vi "滑移力检测.vi"() -> ()   [LabVIEW 2020]
uses:
  <vilib>/Utility/miscctls.llb/LVRowAndColumnTypeDef.ctl
  Global_Variable/Global.vi
  Global_Variable/A131258.vi
  Database/Global1.vi
  <vilib>/addons/database/Connection.llb/DB Tools Open Connec (String).vi
  <vilib>/addons/database/Connection.llb/Conn Execute.vi
  <vilib>/addons/database/Recordset.llb/Rec Fetch Recordset Data (R).vi
  <vilib>/Utility/config.llb/NI_LVConfig.lvlib
  <vilib>/addons/database/NI_Database_API.lvlib
panel:
  out "最大值下限":dbl format="%_4g"
  out "最大值上限":dbl format="%_4g"
  out "拉位移内最大压力(N)":dbl format="%_5g"
  out "压位移内最大压力(N)":dbl format="%_5g"
  out "上序状态显示":string
  out "上序状态":bool
  out "产品追溯码":string
  in  "质量报警":bool
  in  "设备缺料":bool
  in  "设备故障":bool
  out "USER_ID":string
  out "产品型号":string
  out "联机模式":string
  out "用户权限":string
  out "用户名":string
  in  "报表":string[][](table)=[["mm"], ["mm/s"]]
  in  "判定结果 3":bool[][](array[boolean])=[[TRUE]]
  out "拉力判定框内波动压力(N)":dbl format="%_5g"
  out "压力判定框内波动压力(N)":dbl format="%_5g"
  in  "选项卡控件 2":enum32{"滑移力曲线", "参数查看"}(tab)
  out "力位移曲线 3":cluster{dbl[], dbl[]}[](graph)
  out "压位移内最小压力(N)":dbl format="%_5g"
  out "拉位移内最小压力(N)":dbl format="%_5g"
  out "最小值上限":dbl format="%_4g"
  out "最小值下限":dbl format="%_4g"
  in  "产品型号":string(combo)
  in  "选项卡控件 3":enum32{"工位参数", "产品管理", "用户管理"}(tab)
  in  "启用最小值":bool
  in  "坐标轴参数":string[][](table)=[["mm"], ["mm/s"]]
  in  "判定框参数":string[][](table)=[["mm"], ["mm/s"]]
  in  "结果判定参数":string[][](table)=[["mm"], ["mm/s"]]
  in  "删除":bool
  in  "确定":bool
  in  "添加":bool
  in  "退出":bool
  in  "更新":bool
  in  "请输入添加的产品名称":string
  in  "请选择要删除的产品":string(combo)
  in  "进入用户管理":bool
  out "deviceid":string
  out "Fdeviceid":string
  out "codeid":string
  out "productid":string
  out "产品追溯码 2":string
  # "上序状态："
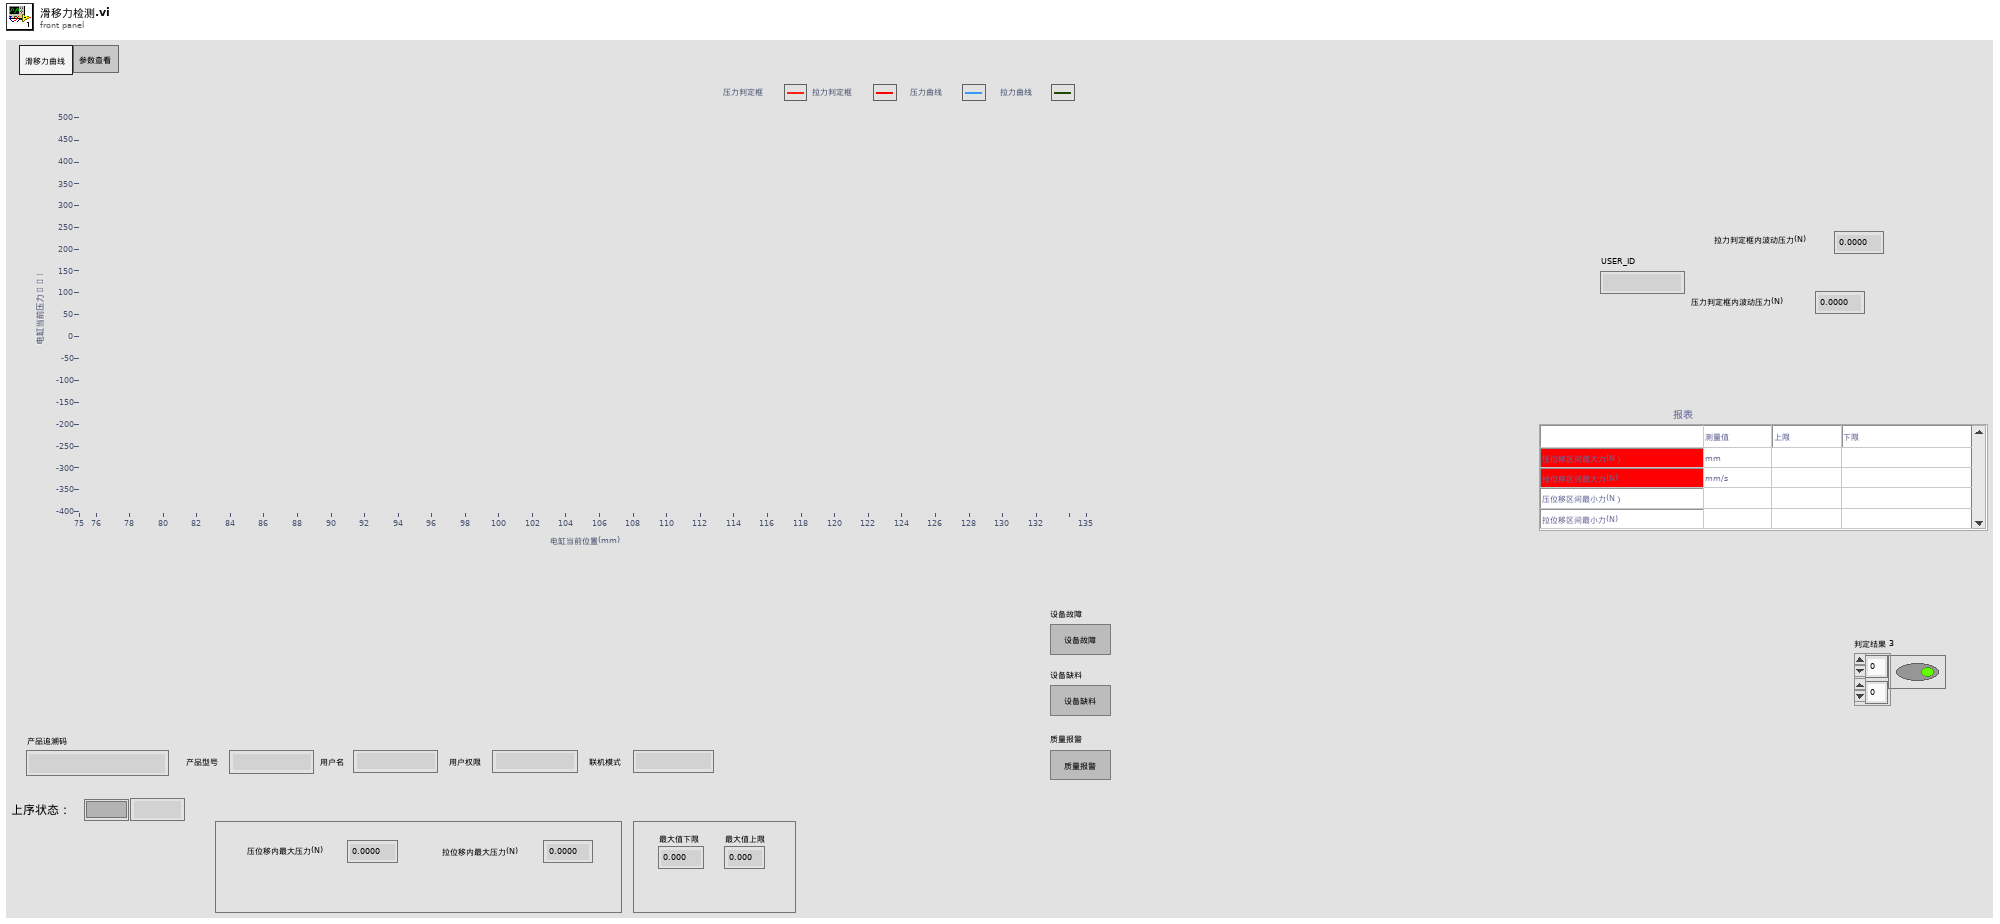
[diagram p1: front panel]
types:
  T1 = enum32{"Invalid", "Standard", "Closed", "Hidden", "Minimized", "Maximized"}
  T2 = typedef "LVRowAndColumnTypeDef.ctl" = cluster{"Row":i32, "Column":i32}
  T3 = cluster{"用户编号":string, "用户名":string, "用户密码(密文)":string, "用户权限":string}
  T4 = cluster{"设备名称":string, "用户名":string, "设备状态":enum16{"设备离线", "设备正常", "设备缺料", "设备故障", "质量报警"}, "附加信息":string}
  T5 = typedef "NI_LVConfig.lvlib/Config Data RefNum.ctl" = refnum<k1>
  T6 = cluster{"输入旋转位移":sgl, "电缸位移":sgl, "工装移载位移":sgl, "输入编码位移":sgl, "输入扭矩":sgl, "123":sgl, "拉压力":sgl, "吸收电流":sgl}
  T7 = cluster{"测试范围":cluster{"单位":string, "下限":dbl, "上限":dbl}, "压力测试最大值":cluster{"单位":string, "下限":dbl, "上限":dbl}, "拉力测试最大值":cluster{"单位":string, "下限":dbl, "上限":dbl}}
  T8 = cluster{"测试范围":cluster{"单位":string, "下限":dbl, "上限":dbl}, "压力测试最大值":cluster{"单位":string, "下限":dbl, "上限":dbl}, "压力测试最小值":cluster{"单位":string, "下限":dbl, "上限":dbl}, "拉力测试最大值":cluster{"单位":string, "下限":dbl, "上限":dbl}, "拉力判定最小值":cluster{"单位":string, "下限":dbl, "上限":dbl}}
  T9 = typedef "NI_Database_API.lvlib/Conn ObjectReference.ctl" = refnum<k1>
  T10 = typedef "NI_Database_API.lvlib/Rec ObjectReference.ctl" = refnum<k1>
  T11 = cluster{"[0]":cluster{string, dbl, dbl}, "[1]":cluster{string, dbl, dbl}, "[2]":cluster{string, dbl, dbl}, "[3]":cluster{string, dbl, dbl}, "[4]":cluster{string, dbl, dbl}}
  T12 = cluster{"[0]":cluster{string, dbl, dbl}, "[1]":cluster{string, dbl, dbl}, "[2]":cluster{string, dbl, dbl}}
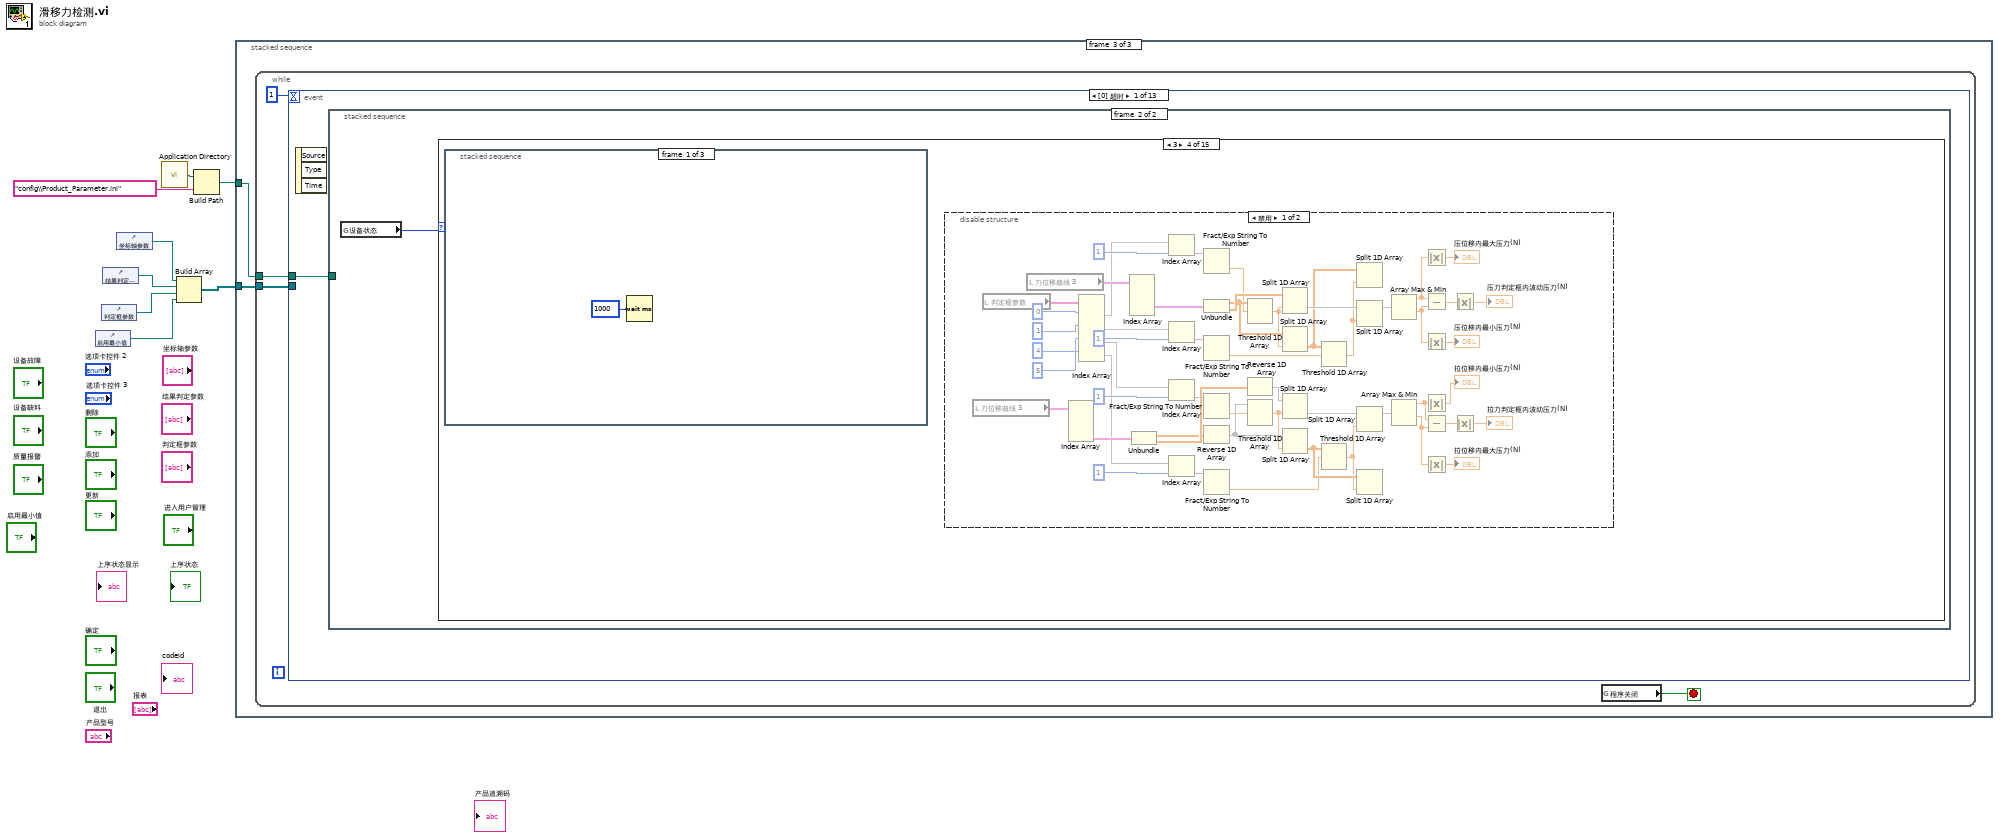
[diagram p0: block diagram]
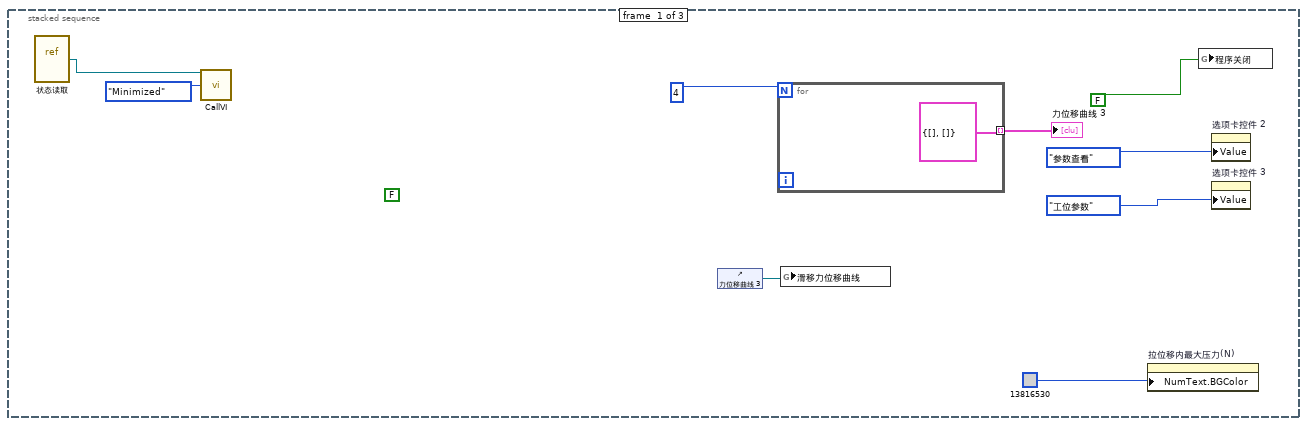
[diagram p2: hidden frame]
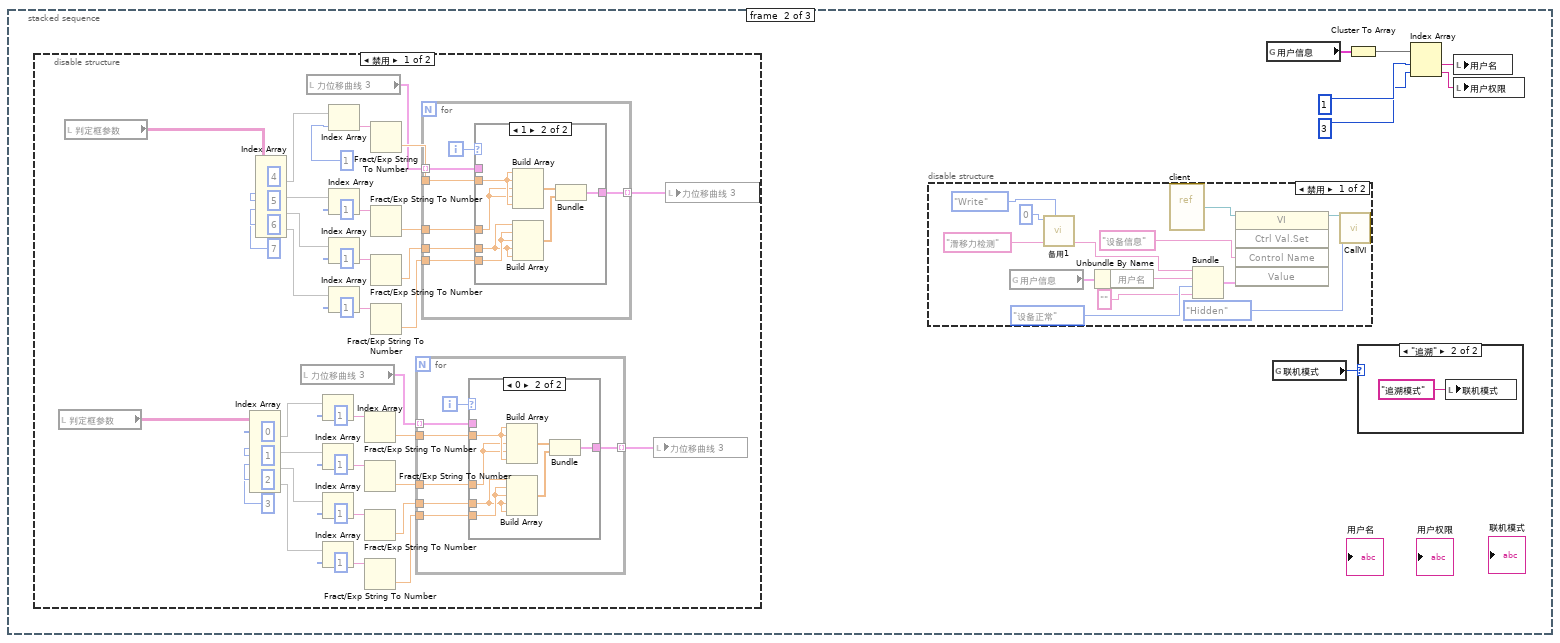
[diagram p3: hidden frame]
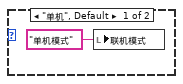
[diagram p8: hidden frame]
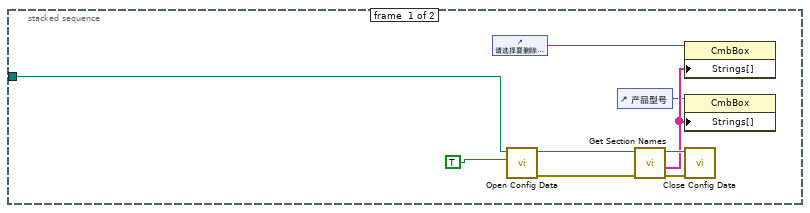
[diagram p9: hidden frame]
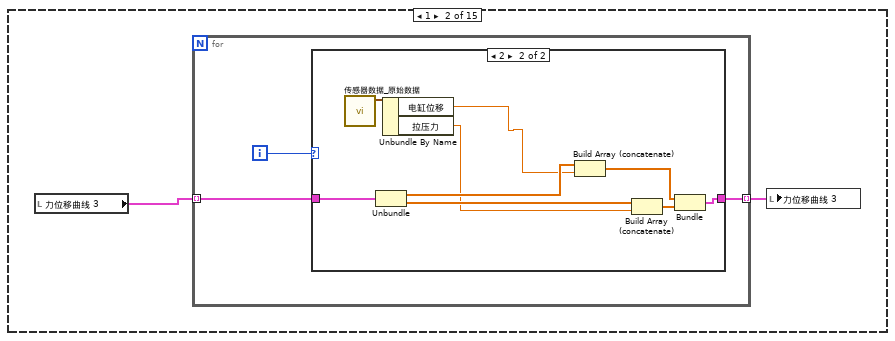
[diagram p11: hidden frame]
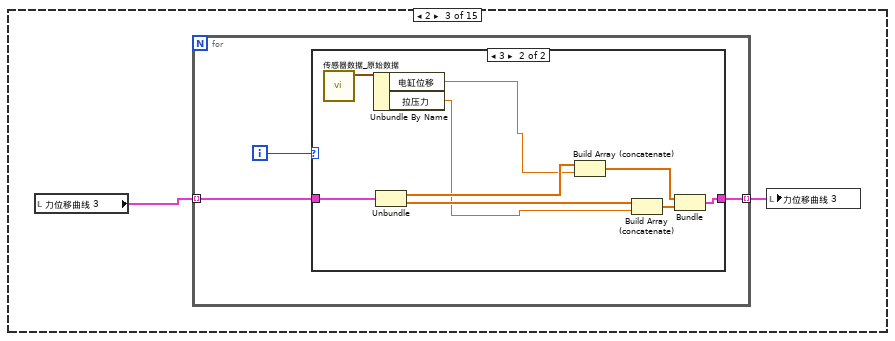
[diagram p13: hidden frame]
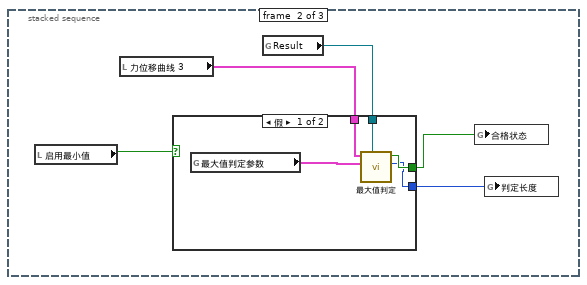
[diagram p15: hidden frame]
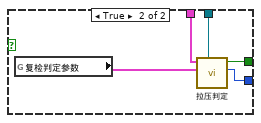
[diagram p16: hidden frame]
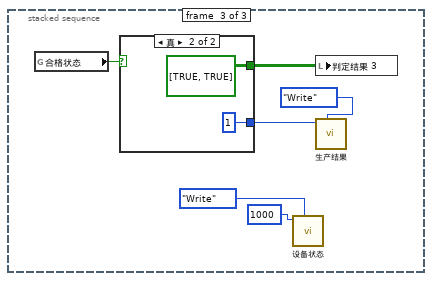
[diagram p17: hidden frame]
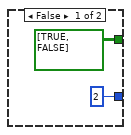
[diagram p18: hidden frame]
diagram:
  n1 = control-ref of="启用最小值"() -> (w1:refnum<vi>)
  n2 = control-ref of="判定框参数"() -> (w2:refnum<vi>)
  n3 = control-ref of="结果判定参数"() -> (w3:refnum<vi>)
  n4 = control-ref of="坐标轴参数"() -> (w4:refnum<vi>)
  n5 = call <vilib>:"Application Directory.vi"() -> ("Application Directory"=w8:path)
  n6 = Build Array(w4, w3, w2, w1) -> (w5:refnum<vi>[])
  n7 = Build Path(base path=w8, name or relative path="config\\Product_Parameter.ini" ("名称或相对路径")) -> (appended path=w6:path)
  n8 = stacked-sequence {
    tunnel: w6 -> [_ _ w117]
    tunnel: w5 -> [_ _ w116]
    frame #0 {
      (unwired) FALSE ("值(信号)")
      n9 = vi-ref "状态读取.vi"() -> (w11:refnum<vi>)
      n10 = call "CallVI.vi"("VI引用"=w11, "状态"=T1."Minimized") -> ()  [unwired: 12 in, 2 out]
      n11 = control-ref of="力位移曲线 3"() -> (w9:refnum<vi>)
      n12 = for {
        N: 4 -> [_]
        tunnel: [cluster{dbl[], dbl[]} {[], []}] -> w16 mode=indexing
      }
      "力位移曲线 3" <- w16
      n13 = global write "A131258.vi" "滑移力位移曲线"(w9) -> ()
      n14 = property on="拉位移内最大压力(N)" class="DigNum (严格)"("NumText.BGColor"=u32 13816530) -> ()  [unwired: 2 in, 2 out]
      n15 = global write "Global.vi" "程序关闭"(FALSE ("程序关闭")) -> ()
      n16 = property on="选项卡控件 2" class="TabCtl (严格)"("Value"=enum32{"滑移力曲线", "参数查看"}."参数查看" ("选项卡控件 2")) -> ()  [unwired: 2 in, 2 out]
      n17 = property on="选项卡控件 3" class="TabCtl (严格)"("Value"=enum32{"工位参数", "产品管理"}."工位参数" ("选项卡控件 3")) -> ()  [unwired: 2 in, 2 out]
    }
    frame #1 {
      n18 = disable-structure shown="禁用" {
        frame Disabled {
          n19 = local read "判定框参数"() -> (w38:string[][])
          n20 = local read "判定框参数"() -> (w41:string[][])
          n21 = Index Array(array=w38, index (row) #1=0 ("索引 (行)"), index (row) #2=1 ("索引 (行)"), index (row) #3=2 ("索引 (行)"), index (row) #4=3 ("索引 (行)")) -> (element #1=w79:string[], element #2=w74:string[], element #3=w73:string[], element #4=w72:string[])  [unwired: 4 in]
          n22 = Index Array(array=w41, index (row) #1=4 ("索引 (行)"), index (row) #2=5 ("索引 (行)"), index (row) #3=6 ("索引 (行)"), index (row) #4=7 ("索引 (行)")) -> (element #1=w57:string[], element #2=w52:string[], element #3=w51:string[], element #4=w50:string[])  [unwired: 4 in]
          n23 = local read "力位移曲线 3"() -> (w62:cluster{dbl[], dbl[]}[])
          n24 = local read "力位移曲线 3"() -> (w40:cluster{dbl[], dbl[]}[])
          n25 = Index Array(array=w79, index=1 ("索引")) -> (element=w67:string)
          n26 = Index Array(array=w74, index=1 ("索引")) -> (element=w66:string)
          n27 = Index Array(array=w73, index=1 ("索引")) -> (element=w65:string)
          n28 = Index Array(array=w72, index=1 ("索引")) -> (element=w64:string)
          n29 = Index Array(array=w57, index=1 ("索引")) -> (element=w45:string)
          n30 = Index Array(array=w52, index=1 ("索引")) -> (element=w44:string)
          n31 = Index Array(array=w51, index=1 ("索引")) -> (element=w43:string)
          n32 = Index Array(array=w50, index=1 ("索引")) -> (element=w42:string)
          n33 = Fract/Exp String To Number(string=w67) -> (number=w71:dbl)  [unwired: 3 in, 1 out]
          n34 = Fract/Exp String To Number(string=w66) -> (number=w70:dbl)  [unwired: 3 in, 1 out]
          n35 = Fract/Exp String To Number(string=w65) -> (number=w68:dbl)  [unwired: 3 in, 1 out]
          n36 = Fract/Exp String To Number(string=w64) -> (number=w69:dbl)  [unwired: 3 in, 1 out]
          n37 = Fract/Exp String To Number(string=w45) -> (number=w49:dbl)  [unwired: 3 in, 1 out]
          n38 = Fract/Exp String To Number(string=w44) -> (number=w48:dbl)  [unwired: 3 in, 1 out]
          n39 = Fract/Exp String To Number(string=w43) -> (number=w46:dbl)  [unwired: 3 in, 1 out]
          n40 = Fract/Exp String To Number(string=w42) -> (number=w47:dbl)  [unwired: 3 in, 1 out]
          n41 = for {
            tunnel: [w105] -> w63 mode=indexing
            tunnel: w62 -> [w104] mode=indexing
            tunnel: w71 -> [w102]
            tunnel: w70 -> [w101]
            tunnel: w69 -> [w100]
            tunnel: w68 -> [w99]
            i -> [w103]
            n42 = case shown="0" w103 {
              tunnel: [w106 w111] -> w105
              tunnel: w104 -> [w106 _]
              tunnel: w102 -> [_ w110]
              tunnel: w101 -> [_ w109]
              tunnel: w100 -> [_ w108]
              tunnel: w99 -> [_ w107]
              frame Default {
              }
              frame 0 {
                n43 = Build Array(w110, w110, w109, w109, w110) -> (w112:dbl[])
                n44 = Build Array(w107, w108, w108, w107, w107) -> (w113:dbl[])
                n45 = Bundle(w112, w113) -> (w111:cluster{dbl[], dbl[]})  [unwired: 1 in]
              }
            }
          }
          n46 = for {
            tunnel: [w90] -> w39 mode=indexing
            tunnel: w40 -> [w89] mode=indexing
            tunnel: w49 -> [w87]
            tunnel: w48 -> [w86]
            tunnel: w47 -> [w85]
            tunnel: w46 -> [w84]
            i -> [w88]
            n47 = case shown="1" w88 {
              tunnel: [w91 w96] -> w90
              tunnel: w89 -> [w91 _]
              tunnel: w87 -> [_ w95]
              tunnel: w86 -> [_ w94]
              tunnel: w85 -> [_ w93]
              tunnel: w84 -> [_ w92]
              frame Default {
              }
              frame 1 {
                n48 = Build Array(w95, w95, w94, w94, w95) -> (w97:dbl[])
                n49 = Build Array(w92, w93, w93, w92, w92) -> (w98:dbl[])
                n50 = Bundle(w97, w98) -> (w96:cluster{dbl[], dbl[]})  [unwired: 1 in]
              }
            }
          }
          n51 = local write "力位移曲线 3"(w63) -> ()
          n52 = local write "力位移曲线 3"(w39) -> ()
        }
        frame Enabled {
        }
      }
      n53 = disable-structure shown="禁用" {
        frame Disabled {
          n54 = global read "Global1.vi" "用户信息"() -> (w35:T3)
          n55 = call "备用1.vi"("枚举"=enum16{"Read", "Write"}."Write", "Status_Write"=u16 0 ("备用_1")) -> ()  [unwired: 9 in, 1 out]
          n56 = Unbundle By Name(w35) -> ("用户名"=w36:string)
          n57 = vi-ref "client.vi"() -> (w33:refnum<vi>)
          n58 = Bundle("设备名称"="滑移力检测", "用户名"=w36, "设备状态"=enum16{"设备离线", "设备正常", "设备缺料", "设备故障", "质量报警"}."设备正常", "附加信息"="") -> (w37:T4)  [unwired: 1 in]
          n59 = invoke class="VI" method="Ctrl Val.Set"(reference=w33, "Control Name"="设备信息" ("控件名"), "Value"=w37) -> (reference out=w34:refnum<vi>)  [unwired: 2 in, 4 out]
          n60 = call "CallVI.vi"("VI引用"=w34, "状态"=T1."Hidden") -> ()  [unwired: 12 in, 2 out]
        }
        frame Enabled {
        }
      }
      n61 = global read "Global1.vi" "用户信息"() -> (w25:T3)
      n62 = global read "Global1.vi" "联机模式"() -> (w19:enum16{"单机", "追溯"})
      n63 = Cluster To Array(cluster=w25) -> (array=w24:string[])
      n64 = case shown="\"追溯\"" w19 {
        frame "单机", Default {
          n65 = local write "联机模式"("单机模式" ("联机模式")) -> ()
        }
        frame "追溯" {
          n66 = local write "联机模式"("追溯模式" ("联机模式")) -> ()
        }
      }
      n67 = Index Array(array=w24, index #1=1 ("索引"), index #2=3 ("索引")) -> (element #1=w21:string, element #2=w20:string)
      n68 = local write "用户名"(w21) -> ()
      n69 = local write "用户权限"(w20) -> ()
    }
    frame #2 {
      n70 = while {
        tunnel: w117 -> [w120]
        tunnel: w116 -> [w119]
        stop <- w118 stop-if-true
        n71 = event shown="[0] 超时" {
          selector: _ -> [_ _ _ _ _ _ _ _ _ _ _ _ _]
          dyn-events: _ -> [_ _ _ _ _ _ _ _ _ _ _ _ _]
          timeout: 1 -> [_ _ _ _ _ _ _ _ _ _ _ _ _]
          tunnel: w120 -> [w122 w518 _ w708 w727 _ w738 _ _ _ _ _ _]
          tunnel: w119 -> [_ _ _ w707 w726 _ w737 _ _ _ _ _ _]
          event Timeout {
            n72 = event-data() -> ()  [unwired: 1 in, 3 out]
            n73 = stacked-sequence {
              tunnel: w122 -> [w123 _]
              frame #0 {
                n74 = control-ref of="请选择要删除的产品"() -> (w124:refnum<vi>)
                n75 = call <vilib>:"Open Config Data.vi"("create file if necessary (T)"=TRUE, "configuration file path"=w123) -> ("error out"=w128:errorcluster, "refnum"=w127:T5)  [unwired: 7 in, 1 out]
                n76 = control-ref of="产品型号"() -> (w125:refnum<vi>)
                n77 = call <vilib>:"Get Section Names.vi"("error in (no error)"=w128, "refnum"=w127) -> ("error out"=w130:errorcluster, "section names"=w126:string[], "refnum out"=w129:T5)  [unwired: 7 in]
                n78 = property on="属性节点" class="CmbBox"(reference=w124, "Strings[]"=w126) -> ()  [unwired: 1 in, 2 out]
                n79 = property on="属性节点" class="CmbBox"(reference=w125, "Strings[]"=w126) -> ()  [unwired: 1 in, 2 out]
                n80 = call <vilib>:"Close Config Data.vi"("error in (no error)"=w130, "refnum"=w129) -> ()  [unwired: 8 in, 2 out]
              }
              frame #1 {
                n81 = global read "Global.vi" "设备状态"() -> (w132:i16)
                n82 = case shown="3" w132 {
                  frame 0, Default {
                  }
                  frame 1 {
                    n83 = local read "力位移曲线 3"() -> (w133:cluster{dbl[], dbl[]}[])
                    n84 = for {
                      tunnel: [w137] -> w134 mode=indexing
                      tunnel: w133 -> [w136] mode=indexing
                      i -> [w135]
                      n85 = case shown="2" w135 {
                        tunnel: [w138 w143] -> w137
                        tunnel: w136 -> [w138 w142]
                        frame Default {
                        }
                        frame 2 {
                          n86 = call "传感器数据_原始数据.vi"() -> ("传感器读数"=w141:T6)  [unwired: 11 in]
                          n87 = Unbundle(w142) -> (w147:dbl[], w146:dbl[])
                          n88 = Unbundle By Name(w141) -> ("电缸位移"=w140:sgl, "拉压力"=w139:sgl)
                          n89 = Build Array (concatenate)(w147, w140) -> (w145:dbl[])
                          n90 = Build Array (concatenate)(w146, w139) -> (w144:dbl[])
                          n91 = Bundle(w145, w144) -> (w143:cluster{dbl[], dbl[]})  [unwired: 1 in]
                        }
                      }
                    }
                    n92 = local write "力位移曲线 3"(w134) -> ()
                  }
                  frame 2 {
                    n93 = local read "力位移曲线 3"() -> (w148:cluster{dbl[], dbl[]}[])
                    n94 = for {
                      tunnel: [w152] -> w149 mode=indexing
                      tunnel: w148 -> [w151] mode=indexing
                      i -> [w150]
                      n95 = case shown="3" w150 {
                        tunnel: [w153 w158] -> w152
                        tunnel: w151 -> [w153 w157]
                        frame Default {
                        }
                        frame 3 {
                          n96 = call "传感器数据_原始数据.vi"() -> ("传感器读数"=w156:T6)  [unwired: 11 in]
                          n97 = Unbundle By Name(w156) -> ("电缸位移"=w155:sgl, "拉压力"=w154:sgl)
                          n98 = Unbundle(w157) -> (w162:dbl[], w161:dbl[])
                          n99 = Build Array (concatenate)(w162, w155) -> (w160:dbl[])
                          n100 = Build Array (concatenate)(w161, w154) -> (w159:dbl[])
                          n101 = Bundle(w160, w159) -> (w158:cluster{dbl[], dbl[]})  [unwired: 1 in]
                        }
                      }
                    }
                    n102 = local write "力位移曲线 3"(w149) -> ()
                  }
                  frame 3 {
                    n103 = stacked-sequence {
                      frame #0 {
                        n104 = Wait (ms)(milliseconds to wait=u32 1000 ("等待时间（毫秒）")) -> ()  [unwired: 1 out]
                      }
                      frame #1 {
                        n105 = local read "启用最小值"() -> (w168:bool)
                        n106 = local read "力位移曲线 3"() -> (w167:cluster{dbl[], dbl[]}[])
                        n107 = global read "Global.vi" "Result"() -> (w165:refnum<vi>)
                        n108 = case shown="假" w168 {
                          tunnel: w167 -> [w171 w177]
                          tunnel: w165 -> [w172 w176]
                          tunnel: [w170 w175] -> w164
                          tunnel: [w169 w174] -> w166
                          frame False {
                            n109 = global read "Global.vi" "最大值判定参数"() -> (w173:T7)
                            n110 = call "最大值判定.vi"("Result"=w172, "最大值判定"=w173, "XY曲线"=w171) -> ("大小"=w169:i32, "OK？"=w170:bool)  [unwired: 7 in]
                          }
                          frame True {
                            n111 = global read "Global.vi" "复检判定参数"() -> (w178:T8)
                            n112 = call "拉压判定.vi"("Result"=w176, "判定参数"=w178, "XY曲线"=w177) -> ("大小"=w174:i32, "OK？"=w175:bool)  [unwired: 7 in]
                          }
                        }
                        n113 = global write "Global.vi" "合格状态"(w164) -> ()
                        n114 = global write "Global.vi" "判定长度"(w166) -> ()
                      }
                      frame #2 {
                        n115 = global read "Global.vi" "合格状态"() -> (w184:bool)
                        n116 = case shown="真" w184 {
                          tunnel: [u16 2 ("生产结果") u16 1 ("生产结果")] -> w183
                          tunnel: [bool[][] [[TRUE, FALSE]] ("判定结果") bool[][] [[TRUE, TRUE]] ("判定结果")] -> w182
                          frame False {
                          }
                          frame True {
                          }
                        }
                        n117 = call "设备状态.vi"("枚举"=enum16{"Read", "Write"}."Write", "Status_Write"=u32 1000 ("写入数据")) -> ()  [unwired: 9 in, 1 out]
                        n118 = local write "判定结果 3"(w182) -> ()
                        n119 = call "生产结果.vi"("枚举"=enum16{"Read", "Write"}."Write", "Status_Write"=w183) -> ()  [unwired: 9 in, 1 out]
                      }
                    }
                    n120 = disable-structure shown="禁用" {
                      frame Disabled {
                        n121 = local read "力位移曲线 3"() -> (w233:cluster{dbl[], dbl[]}[])
                        n122 = local read "判定框参数"() -> (w201:string[][])
                        n123 = local read "力位移曲线 3"() -> (w241:cluster{dbl[], dbl[]}[])
                        n124 = Index Array(array=w233) -> (element #4=w226:cluster{dbl[], dbl[]})  [unwired: 4 in, 3 out]
                        n125 = Index Array(array=w201, index (row) #1=0 ("索引 (行)"), index (row) #2=1 ("索引 (行)"), index (row) #3=4 ("索引 (行)"), index (row) #4=5 ("索引 (行)")) -> (element #1=w193:string[], element #2=w194:string[], element #3=w195:string[], element #4=w196:string[])  [unwired: 4 in]
                        n126 = Index Array(array=w241) -> (element #3=w227:cluster{dbl[], dbl[]})  [unwired: 4 in, 3 out]
                        n127 = Unbundle(w226) -> (w211:dbl[], w213:dbl[])
                        n128 = Index Array(array=w193, index=1 ("索引")) -> (element=w197:string)
                        n129 = Index Array(array=w194, index=1 ("索引")) -> (element=w198:string)
                        n130 = Index Array(array=w195, index=1 ("索引")) -> (element=w199:string)
                        n131 = Index Array(array=w196, index=1 ("索引")) -> (element=w200:string)
                        n132 = Fract/Exp String To Number(string=w197) -> (number=w192:dbl)  [unwired: 3 in, 1 out]
                        n133 = Unbundle(w227) -> (w239:dbl[], w240:dbl[])
                        n134 = Fract/Exp String To Number(string=w198) -> (number=w191:dbl)  [unwired: 3 in, 1 out]
                        n135 = Fract/Exp String To Number(string=w199) -> (number=w190:dbl)  [unwired: 3 in, 1 out]
                        n136 = Reverse 1D Array(array=w211) -> (reversed array=w210:dbl[])
                        n137 = Fract/Exp String To Number(string=w200) -> (number=w189:dbl)  [unwired: 3 in, 1 out]
                        n138 = Threshold 1D Array(2:w192, 3:w239) -> (0:w238:dbl)  [unwired: 1 in]
                        n139 = Reverse 1D Array(array=w213) -> (reversed array=w212:dbl[])
                        n140 = Threshold 1D Array(2:w190, 3:w210) -> (0:w232:dbl)  [unwired: 1 in]
                        n141 = Split 1D Array(array=w240, index=w238) -> (second subarray=w237:dbl[])  [unwired: 1 out]
                        n142 = Split 1D Array(array=w239, index=w238) -> (second subarray=w236:dbl[])  [unwired: 1 out]
                        n143 = Split 1D Array(array=w212, index=w232) -> (second subarray=w231:dbl[])  [unwired: 1 out]
                        n144 = Split 1D Array(array=w210, index=w232) -> (second subarray=w230:dbl[])  [unwired: 1 out]
                        n145 = Threshold 1D Array(2:w191, 3:w236) -> (0:w235:dbl)  [unwired: 1 in]
                        n146 = Threshold 1D Array(2:w189, 3:w230) -> (0:w229:dbl)  [unwired: 1 in]
                        n147 = Split 1D Array(array=w236, index=w235) -> ()  [unwired: 2 out]
                        n148 = Split 1D Array(array=w237, index=w235) -> (first subarray=w234:dbl[])  [unwired: 1 out]
                        n149 = Split 1D Array(array=w231, index=w229) -> (first subarray=w228:dbl[])  [unwired: 1 out]
                        n150 = Split 1D Array(array=w230, index=w229) -> ()  [unwired: 2 out]
                        n151 = Array Max & Min(array=w234) -> (max value=w217:dbl, min value=w215:dbl)  [unwired: 2 out]
                        n152 = Array Max & Min(array=w228) -> (max value=w225:dbl, min value=w223:dbl)  [unwired: 2 out]
                        n153 = Absolute Value(x=w217) -> (abs(x)=→"压位移内最大压力(N)":dbl)
                        n154 = Subtract(x=w217, y=w215) -> (x-y=w219:dbl)
                        n155 = Absolute Value(x=w215) -> (abs(x)=→"压位移内最小压力(N)":dbl)
                        n156 = Absolute Value(x=w225) -> (abs(x)=→"拉位移内最小压力(N)":dbl)
                        n157 = Subtract(x=w225, y=w223) -> (x-y=w221:dbl)
                        n158 = Absolute Value(x=w223) -> (abs(x)=→"拉位移内最大压力(N)":dbl)
                        n159 = Absolute Value(x=w219) -> (abs(x)=→"压力判定框内波动压力(N)":dbl)
                        n160 = Absolute Value(x=w221) -> (abs(x)=→"拉力判定框内波动压力(N)":dbl)
                      }
                      frame Enabled {
                      }
                    }
                  }
                  frame 8 {
                  }
                  frame 4 {
                    n161 = stacked-sequence {
                      frame #0 {
                        w243 = u32 13816530
                        (unwired) FALSE ("不合格指示灯")
                        (unwired) FALSE ("合格指示灯")
                        w244 = 0
                        n162 = local write "压力判定框内波动压力(N)"(w244) -> ()
                        n163 = local write "拉力判定框内波动压力(N)"(w244) -> ()
                        n164 = local write "压位移内最大压力(N)"(w244) -> ()
                        n165 = local write "压位移内最小压力(N)"(w244) -> ()
                        n166 = local write "拉位移内最小压力(N)"(w244) -> ()
                        n167 = local write "拉位移内最大压力(N)"(w244) -> ()
                        n168 = Wait (ms)(milliseconds to wait=u32 500 ("等待时间（毫秒）")) -> ()  [unwired: 1 out]
                        n169 = property on="压位移内最小压力(N)" class="DigNum (严格)"("NumText.BGColor"=w243) -> ()  [unwired: 2 in, 2 out]
                        n170 = property on="拉位移内最小压力(N)" class="DigNum (严格)"("NumText.BGColor"=w243) -> ()  [unwired: 2 in, 2 out]
                        n171 = property on="拉位移内最大压力(N)" class="DigNum (严格)"("NumText.BGColor"=w243) -> ()  [unwired: 2 in, 2 out]
                        n172 = property on="压位移内最大压力(N)" class="DigNum (严格)"("NumText.BGColor"=w243) -> ()  [unwired: 2 in, 2 out]
                        n173 = for {
                          N: 4 -> [_]
                          tunnel: [cluster{dbl[], dbl[]} {[], []}] -> w246 mode=indexing
                        }
                        n174 = local write "力位移曲线 3"(w246) -> ()
                      }
                      frame #1 {
                        n175 = global read "Global.vi" "Result"() -> (w254:refnum<vi>)
                        n176 = property class="Tbl"(reference=w254, "Row Headers[]"=string[] [] ("行首字符串[]")) -> (reference out=w252:refnum<vi>)  [unwired: 1 in, 1 out]
                        n177 = property class="Tbl"(reference=w252, "Value"=string[][] [] ("值")) -> (reference out=w250:refnum<vi>)  [unwired: 1 in, 1 out]
                        n178 = property class="Tbl"(reference=w250, "Active Cell"=T2 {"Row"=-2, "Column"=-2} ("活动单元格:活动单元格"), "Cell BG Color"=u32 16777216 ("活动单元格:单元格背景色")) -> ()  [unwired: 1 in, 2 out]
                        n179 = call "设备状态.vi"("枚举"=enum16{"Read", "Write"}."Write", "Status_Write"=5) -> ()  [unwired: 9 in, 1 out]
                        n180 = call "生产结果.vi"("枚举"=enum16{"Read", "Write"}."Write", "Status_Write"=u16 0 ("生产结果")) -> ()  [unwired: 9 in, 1 out]
                      }
                    }
                  }
                  frame 5 {
                    w260 = u16 0 ("备用_1")
                    n181 = call "备用1.vi"("枚举"=enum16{"Read", "Write"}."Write", "Status_Write"=w260) -> ()  [unwired: 9 in, 1 out]
                    n182 = call "设备状态.vi"("Status_Write"=w260) -> ()  [unwired: 10 in, 1 out]
                    n183 = local read "力位移曲线 3"() -> (w262:cluster{dbl[], dbl[]}[])
                    n184 = for {
                      tunnel: [w265] -> w261 mode=indexing
                      tunnel: w262 -> [w264] mode=indexing
                      i -> [w263]
                      n185 = case shown="1" w263 {
                        tunnel: [w266 w288 w291] -> w265
                        tunnel: w264 -> [w266 _ _]
                        frame Default {
                        }
                        frame 0 {
                          n186 = local read "判定框参数"() -> (w279:string[][])
                          n187 = Index Array(array=w279, index (row) #1=0 ("索引 (行)"), index (row) #2=0 ("索引 (行)"), index (row) #3=1 ("索引 (行)"), index (row) #4=1 ("索引 (行)")) -> (element #1=w271:string[], element #2=w272:string[], element #3=w273:string[], element #4=w274:string[])  [unwired: 4 in]
                          n188 = Index Array(array=w271, index=1 ("索引")) -> (element=w275:string)
                          n189 = Index Array(array=w272, index=2 ("索引")) -> (element=w276:string)
                          n190 = Index Array(array=w273, index=1 ("索引")) -> (element=w277:string)
                          n191 = Index Array(array=w274, index=2 ("索引")) -> (element=w278:string)
                          n192 = Fract/Exp String To Number(string=w275) -> (number=w269:dbl)  [unwired: 3 in, 1 out]
                          n193 = Fract/Exp String To Number(string=w276) -> (number=w270:dbl)  [unwired: 3 in, 1 out]
                          n194 = Fract/Exp String To Number(string=w277) -> (number=w268:dbl)  [unwired: 3 in, 1 out]
                          n195 = Fract/Exp String To Number(string=w278) -> (number=w267:dbl)  [unwired: 3 in, 1 out]
                          n196 = Build Array(w270, w270, w269, w269, w270) -> (w289:dbl[])
                          n197 = Build Array(w267, w268, w268, w267, w267) -> (w290:dbl[])
                          n198 = Bundle(w289, w290) -> (w288:cluster{dbl[], dbl[]})  [unwired: 1 in]
                        }
                        frame 1 {
                          n199 = local read "判定框参数"() -> (w312:string[][])
                          n200 = Index Array(array=w312, index (row) #1=2 ("索引 (行)"), index (row) #2=2 ("索引 (行)"), index (row) #3=3 ("索引 (行)"), index (row) #4=3 ("索引 (行)")) -> (element #1=w304:string[], element #2=w305:string[], element #3=w306:string[], element #4=w307:string[])  [unwired: 4 in]
                          n201 = Index Array(array=w304, index=1 ("索引")) -> (element=w308:string)
                          n202 = Index Array(array=w305, index=2 ("索引")) -> (element=w309:string)
                          n203 = Index Array(array=w306, index=1 ("索引")) -> (element=w310:string)
                          n204 = Index Array(array=w307, index=2 ("索引")) -> (element=w311:string)
                          n205 = Fract/Exp String To Number(string=w308) -> (number=w302:dbl)  [unwired: 3 in, 1 out]
                          n206 = Fract/Exp String To Number(string=w309) -> (number=w303:dbl)  [unwired: 3 in, 1 out]
                          n207 = Fract/Exp String To Number(string=w310) -> (number=w301:dbl)  [unwired: 3 in, 1 out]
                          n208 = Fract/Exp String To Number(string=w311) -> (number=w300:dbl)  [unwired: 3 in, 1 out]
                          n209 = Build Array(w303, w303, w302, w302, w303) -> (w313:dbl[])
                          n210 = Build Array(w300, w301, w301, w300, w300) -> (w314:dbl[])
                          n211 = Bundle(w313, w314) -> (w291:cluster{dbl[], dbl[]})  [unwired: 1 in]
                        }
                      }
                    }
                    n212 = local write "力位移曲线 3"(w261) -> ()
                  }
                  frame 101 {
                    w315 = enum16{"Read", "Write"}."Write" ("枚举")
                    w316 = u16 0 ("备用_1")
                    w317 = u32 13816530
                    w318 = 0.0 ("压力判定框内最大压力(N)")
                    (unwired) FALSE ("合格指示灯")
                    n213 = call "生产结果.vi"("枚举"=w315, "Status_Write"=w316) -> ()  [unwired: 9 in, 1 out]
                    n214 = call "备用1.vi"("枚举"=w315, "Status_Write"=w316) -> ()  [unwired: 9 in, 1 out]
                    n215 = local write "压位移内最大压力(N)"(w318) -> ()
                    n216 = local write "压位移内最小压力(N)"(w318) -> ()
                    n217 = local write "压力判定框内波动压力(N)"(w318) -> ()
                    n218 = local write "拉位移内最小压力(N)"(w318) -> ()
                    n219 = local write "拉位移内最大压力(N)"(w318) -> ()
                    n220 = local write "拉力判定框内波动压力(N)"(w318) -> ()
                    n221 = property on="压位移内最大压力(N)" class="DigNum (严格)"("NumText.BGColor"=w317) -> ()  [unwired: 2 in, 2 out]
                    n222 = property on="压位移内最小压力(N)" class="DigNum (严格)"("NumText.BGColor"=w317) -> ()  [unwired: 2 in, 2 out]
                    n223 = property on="拉位移内最小压力(N)" class="DigNum (严格)"("NumText.BGColor"=w317) -> ()  [unwired: 2 in, 2 out]
                    n224 = property on="拉位移内最大压力(N)" class="DigNum (严格)"("NumText.BGColor"=w317) -> ()  [unwired: 2 in, 2 out]
                    n225 = for {
                      N: 4 -> [_]
                      tunnel: [cluster{dbl[], dbl[]} {[], []}] -> w320 mode=indexing
                    }
                    n226 = local write "力位移曲线 3"(w320) -> ()
                  }
                  frame 1000 {
                    w324 = enum16{"Read", "Write"}."Write" ("枚举")
                    n227 = call "浮动通知.vi"("通知内容"="报表生成中" ("Status")) -> ()  [unwired: 11 in]
                    n228 = call "设备状态.vi"("枚举"=w324, "Status_Write"=u16 1001 ("拉压力测试状态")) -> ()  [unwired: 9 in, 1 out]
                    n229 = Wait (ms)(milliseconds to wait=u32 100 ("等待时间（毫秒）")) -> ()  [unwired: 1 out]
                    n230 = call "备用1.vi"("枚举"=w324, "Status_Write"=i16 1) -> ()  [unwired: 9 in, 1 out]
                  }
                  frame 1001 {
                    n231 = stacked-sequence {
                      frame #0 {
                        n232 = global read "Global.vi" "产品追溯码"() -> (w327:string)
                        n233 = call "Report_A131258.vi"("文件重命名"=TRUE, "文件名称"=w327, "布尔数组"="判定结果 3") -> ()  [unwired: 8 in, 1 out]
                      }
                      frame #1 {
                        n234 = Wait (ms)(milliseconds to wait=u32 200 ("等待时间（毫秒）")) -> ()  [unwired: 1 out]
                        n235 = call "设备状态.vi"("枚举"=enum16{"Read", "Write"}."Write", "Status_Write"=i16 1002) -> ()  [unwired: 9 in, 1 out]
                      }
                    }
                  }
                  frame 1002 {
                    n236 = global read "Global1.vi" "联机模式"() -> (w333:enum16{"单机", "追溯"})
                    n237 = case shown="\"追溯\"" w333 {
                      tunnel: w333 -> [_ w337]
                      frame "单机", Default {
                        n238 = call "设备状态.vi"("枚举"=enum16{"Read", "Write"}."Write", "Status_Write"=i16 1003) -> ()  [unwired: 9 in, 1 out]
                        n239 = disable-structure shown="禁用" {
                          frame Disabled {
                            n240 = shared-variable "我的电脑\\200滑移力曲线.lvlib\\拉压力测试状态"(u16 1003 ("备用1")) -> ()  [unwired: 1 in, 1 out]
                          }
                          frame Enabled {
                          }
                        }
                      }
                      frame "追溯" {
                        n241 = stacked-sequence {
                          tunnel: w337 -> [w338 _]
                          frame #0 {
                            n242 = case shown="\"追溯\"" w338 {
                              frame "单机", Default {
                              }
                              frame "追溯" {
                                n243 = global read "Global.vi" "Result"() -> (w348:refnum<vi>)
                                n244 = property class="Tbl"(reference=w348) -> (reference out=w347:refnum<vi>, "Row Headers[]"=w346:string[])  [unwired: 1 in, 1 out]
                                n245 = property class="Tbl"(reference=w347) -> ("Value"=w345:string[][])  [unwired: 1 in, 2 out]
                                n246 = call "浮动通知.vi"("通知内容"="数据上传") -> ()  [unwired: 11 in]
                                n247 = for {
                                tunnel: w346 -> [w353] mode=indexing
                                tunnel: w345 -> [w352] mode=indexing
                                tunnel: [w350] -> w340 mode=indexing if=w349
                                n248 = Build Array (concatenate)(w353, w352) -> (w350:string[])
                                n249 = Index Array(array=w352) -> (element=w351:string)  [unwired: 1 in]
                                n250 = case shown="\"\"" w351 {
                                tunnel: [TRUE FALSE] -> w349
                                frame Default {
                                }
                                frame "" {
                                }
                                }
                                }
                                n251 = global read "追溯全部变量.vi" "工件状态"() -> (w344:string)
                                n252 = local read "deviceid"() -> (w342:string)
                                n253 = local read "USER_ID"() -> (w343:string)
                                n254 = local read "codeid"() -> (w341:string)
                                n255 = call "UPRESULT.vi"("DEVICE_ID"=w342, "USER_ID"=w343, "CODE_ID"=w341, "RESULT_VALUE"=w344) -> ()  [unwired: 11 in, 1 out]
                                n256 = call "UPTEST.vi"("Result"=w340, "CODE_ID"=w341, "DEVICE_ID"=w342) -> ()  [unwired: 6 in, 1 out]
                              }
                            }
                          }
                          frame #1 {
                            n257 = call "设备状态.vi"("枚举"=enum16{"Read", "Write"}."Write", "Status_Write"=i16 1003) -> ()  [unwired: 9 in, 1 out]
                            n258 = disable-structure shown="禁用" {
                              frame Disabled {
                                n259 = shared-variable "我的电脑\\200滑移力曲线.lvlib\\拉压力测试状态"(u16 1003 ("备用1")) -> ()  [unwired: 1 in, 1 out]
                              }
                              frame Enabled {
                              }
                            }
                          }
                        }
                      }
                    }
                  }
                  frame 1003 {
                    n260 = global read "Global1.vi" "联机模式"() -> (w359:enum16{"单机", "追溯"})
                    n261 = case shown="\"单机\", 默认" w359 {
                      tunnel: w359 -> [_ _]
                      frame "单机", Default {
                        n262 = disable-structure shown="禁用" {
                          frame Disabled {
                            n263 = shared-variable "我的电脑\\200滑移力曲线.lvlib\\拉压力测试状态"(u16 0 ("备用1")) -> ()  [unwired: 1 in, 1 out]
                            n264 = shared-variable "我的电脑\\200滑移力曲线.lvlib\\备用_1"(u16 0 ("备用_1")) -> ()  [unwired: 1 in, 1 out]
                          }
                          frame Enabled {
                          }
                        }
                        n265 = call "备用1.vi"("枚举"=enum16{"Read", "Write"}."Write", "Status_Write"=i16 0) -> ()  [unwired: 9 in, 1 out]
                        n266 = call "设备状态.vi"("枚举"=enum16{"Read", "Write"}."Write", "Status_Write"=u16 0 ("备用1")) -> ()  [unwired: 9 in, 1 out]
                      }
                      frame "追溯" {
                        w368 = enum16{"Read", "Write"}."Write" ("枚举")
                        n267 = disable-structure shown="禁用" {
                          frame Disabled {
                            n268 = shared-variable "我的电脑\\200滑移力曲线.lvlib\\拉压力测试状态"(u16 0 ("备用1")) -> ()  [unwired: 1 in, 1 out]
                            n269 = shared-variable "我的电脑\\200滑移力曲线.lvlib\\备用_1"(u16 0 ("备用_1")) -> ()  [unwired: 1 in, 1 out]
                          }
                          frame Enabled {
                          }
                        }
                        n270 = call "设备状态.vi"("枚举"=w368, "Status_Write"=i16 0) -> ()  [unwired: 9 in, 1 out]
                        n271 = call "备用1.vi"("枚举"=w368, "Status_Write"=i16 0) -> ()  [unwired: 9 in, 1 out]
                      }
                    }
                  }
                  frame 2000 {
                    n272 = stacked-sequence {
                      frame #0 {
                        n273 = Wait (ms)(milliseconds to wait=u32 300 ("等待时间（毫秒）")) -> ()  [unwired: 1 out]
                        n274 = global write "Global.vi" "判定长度"(0 ("判定长度")) -> ()
                        n275 = global write "Global.vi" "产品追溯码"("" ("产品追溯码")) -> ()
                        n276 = local write "判定结果 3"(bool[][] [] ("判定结果 3")) -> ()
                      }
                      frame #1 {
                        w378 = "" ("上序状态显示")
                        w383 = "请扫码！" ("通知内容")
                        n277 = global read "Global.vi" "上序状态颜色"() -> (w379:refnum<vi>)
                        n278 = property class="Str"(reference=w379, "Value"=w378) -> (reference out=w377:refnum<vi>)  [unwired: 1 in, 1 out]
                        n279 = property class="Str"(reference=w377, "Text.BGColor"=u32 16777216) -> ()  [unwired: 1 in, 2 out]
                        n280 = local write "上序状态显示"(w378) -> ()
                        n281 = call "浮动通知.vi"("通知内容"=w383) -> ()  [unwired: 11 in]
                        n282 = property on="上序状态" class="Bool (严格)"("Colors [4]"=cluster{u32, u32}[] [{11776947, 11776947}, {11776947, 11776947}, {11776947, 11776947}, {11776947, 11776947}]) -> ()  [unwired: 2 in, 2 out]
                        n283 = call "输入框.vi"("提示信息"=w383) -> ("条形码输出"=w375:string)
                        n284 = global write "Global.vi" "产品追溯码"(w375) -> ()
                        n285 = call "设备状态.vi"("枚举"=enum16{"Read", "Write"}."Write", "Status_Write"=i16 2001) -> ()  [unwired: 9 in, 1 out]
                      }
                    }
                  }
                  frame 2001 {
                    n286 = global read "Global.vi" "产品追溯码"() -> (w384:string)
                    n287 = String Length(string=w384) -> (length=w386:i32)
                    n288 = Greater?(x=w386, y=4) -> (0:w387:bool)
                    n289 = case shown="真" w387 {
                      frame False {
                      }
                      frame True {
                        n290 = call "设备状态.vi"("枚举"=enum16{"Read", "Write"}."Write", "Status_Write"=i16 2100) -> ()  [unwired: 9 in, 1 out]
                      }
                    }
                  }
                  frame 2100 {
                    n291 = global read "Global1.vi" "联机模式"() -> (w390:enum16{"单机", "追溯"})
                    n292 = case shown="\"追溯\"" w390 {
                      selector: w390 -> [_ w397]
                      frame "单机", Default {
                        n293 = disable-structure shown="禁用" {
                          frame Disabled {
                            n294 = shared-variable "我的电脑\\200滑移力曲线.lvlib\\拉压力测试状态"(u16 2002 ("备用1")) -> ()  [unwired: 1 in, 1 out]
                          }
                          frame Enabled {
                          }
                        }
                        n295 = call "设备状态.vi"("枚举"=enum16{"Read", "Write"}."Write", "Status_Write"=i16 2002) -> ()  [unwired: 9 in, 1 out]
                      }
                      frame "追溯" {
                        n296 = local read "Fdeviceid"() -> (w396:string)
                        n297 = Equal?(x=w396, y="") -> (x = y?=w395:bool)
                        n298 = case shown="假" w395 {
                          tunnel: w397 -> [w398 w466]
                          frame False {
                            n299 = stacked-sequence {
                              tunnel: w398 -> [_ _]
                              frame #0 {
                                n300 = global read "Global.vi" "产品追溯码"() -> (w399:string)
                                n301 = local read "productid"() -> (w407:string)
                                n302 = global read "Global1.vi" "联机模式"() -> (w420:enum16{"单机", "追溯"})
                                n303 = call "GetSQLstring.vi"("联机模式"=w420) -> ("错误输出"=w418:errorcluster, "连接字符串"=w419:string)  [unwired: 9 in]
                                n304 = Concatenate Strings("SELECT CODE_ID  FROM CODE  WHERE CODE_SENSOR ='" ("字符串"), w399, "'" ("字符串"), " AND PRODUCT_ID='" ("字符串"), w407, "'" ("字符串")) -> (w417:string)
                                n305 = call-poly <vilib>:"DB Tools Open Connection.vi"("error in (no error)"=w418, "connection information"=w419) -> ("error out"=w412:errorcluster, "connection reference"=w413:T9)  [unwired: 6 in]
                                n306 = call-poly <vilib>:"DB Tools Execute Query.vi"("error in (no error)"=w412, "SQL query"=w417, "connection reference"=w413) -> ("error out"=w415:errorcluster, "recordset reference"=w416:T10)  [unwired: 5 in]
                                n307 = call-poly <vilib>:"DB Tools Fetch Recordset Data.vi"("error in (no error)"=w415, "recordset reference"=w416) -> ("error out"=w411:errorcluster, "recordset data"=w414:variant[][])  [unwired: 3 in, 1 out]
                                n308 = Variant To Data(error in=w411, type=string[][] [], Variant=w414) -> (data=w410:string[][])  [unwired: 1 out]
                                n309 = Index Array(array=w410, index (row)=0 ("索引 (行)")) -> (element=w409:string[])  [unwired: 1 in]
                                n310 = Index Array(array=w409, index=0 ("索引 (行)")) -> (element=w408:string)
                                n311 = local write "codeid"(w408) -> ()
                              }
                              frame #1 {
                                n312 = local read "Fdeviceid"() -> (w427:string)
                                n313 = global read "Global1.vi" "联机模式"() -> (w441:enum16{"单机", "追溯"})
                                n314 = local read "codeid"() -> (w429:string)
                                n315 = call "GetSQLstring.vi"("联机模式"=w441) -> ("错误输出"=w439:errorcluster, "连接字符串"=w440:string)  [unwired: 9 in]
                                n316 = Concatenate Strings("SELECT RESULT_VALUE FROM RESULT  WHERE DEVICE_ID =\n" ("table"), w427, " AND CODE_ID ='" ("字符串"), w429, "'" ("字符串")) -> (w438:string)
                                n317 = call-poly <vilib>:"DB Tools Open Connection.vi"("error in (no error)"=w439, "connection information"=w440) -> ("error out"=w433:errorcluster, "connection reference"=w434:T9)  [unwired: 6 in]
                                n318 = call-poly <vilib>:"DB Tools Execute Query.vi"("error in (no error)"=w433, "SQL query"=w438, "connection reference"=w434) -> ("error out"=w436:errorcluster, "recordset reference"=w437:T10)  [unwired: 5 in]
                                n319 = call-poly <vilib>:"DB Tools Fetch Recordset Data.vi"("error in (no error)"=w436, "recordset reference"=w437) -> ("error out"=w432:errorcluster, "recordset data"=w435:variant[][])  [unwired: 3 in, 1 out]
                                n320 = Variant To Data(error in=w432, type=string[][] [], Variant=w435) -> (data=w430:string[][])  [unwired: 1 out]
                                n321 = Index Array(array=w430, index (row)=0 ("索引 (行)")) -> (element=w431:string[])  [unwired: 1 in]
                                n322 = Index Array(array=w431, index=0 ("索引 (行)")) -> (element=w428:string)
                                n323 = case shown="\"\"" w428 {
                                frame "假", Default {
                                }
                                frame "" {
                                n324 = global read "Global.vi" "上序状态颜色"() -> (w445:refnum<vi>)
                                n325 = local write "上序状态显示"("漏序" ("上序状态显示")) -> ()
                                n326 = property class="Str"(reference=w445, "Value"="漏序" ("上序状态显示")) -> (reference out=w443:refnum<vi>)  [unwired: 1 in, 1 out]
                                n327 = property on="上序状态" class="Bool (严格)"("Colors [4]"=cluster{u32, u32}[] [{16767232, 16767232}, {16767232, 16767232}, {16767232, 16767232}, {16767232, 16767232}]) -> ()  [unwired: 2 in, 2 out]
                                n328 = property class="Str"(reference=w443, "Text.BGColor"=u32 16767232) -> ()  [unwired: 1 in, 2 out]
                                n329 = call "设备状态.vi"("枚举"=enum16{"Read", "Write"}."Write", "Status_Write"=i16 5000) -> ()  [unwired: 9 in, 1 out]
                                }
                                frame "OK" {
                                n330 = global read "Global.vi" "上序状态颜色"() -> (w453:refnum<vi>)
                                n331 = local write "上序状态显示"("合格" ("上序状态显示")) -> ()
                                n332 = property class="Str"(reference=w453, "Value"="合格" ("上序状态显示")) -> (reference out=w451:refnum<vi>)  [unwired: 1 in, 1 out]
                                n333 = property on="上序状态" class="Bool (严格)"("Colors [4]"=cluster{u32, u32}[] [{6618880, 6618880}, {6618880, 6618880}, {6618880, 6618880}, {6618880, 6618880}]) -> ()  [unwired: 2 in, 2 out]
                                n334 = property class="Str"(reference=w451, "Text.BGColor"=u32 6618880) -> ()  [unwired: 1 in, 2 out]
                                n335 = call "设备状态.vi"("枚举"=enum16{"Read", "Write"}."Write", "Status_Write"=i16 2002) -> ()  [unwired: 9 in, 1 out]
                                }
                                frame "NG" {
                                n336 = global read "Global.vi" "上序状态颜色"() -> (w461:refnum<vi>)
                                n337 = local write "上序状态显示"("不合格" ("上序状态显示")) -> ()
                                n338 = property class="Str"(reference=w461, "Value"="不合格" ("上序状态显示")) -> (reference out=w459:refnum<vi>)  [unwired: 1 in, 1 out]
                                n339 = property on="上序状态" class="Bool (严格)"("Colors [4]"=cluster{u32, u32}[] [{16711680, 16711680}, {16711680, 16711680}, {16711680, 16711680}, {16711680, 16711680}]) -> ()  [unwired: 2 in, 2 out]
                                n340 = property class="Str"(reference=w459, "Text.BGColor"=u32 16711680) -> ()  [unwired: 1 in, 2 out]
                                n341 = call "设备状态.vi"("枚举"=enum16{"Read", "Write"}."Write", "Status_Write"=i16 5000) -> ()  [unwired: 9 in, 1 out]
                                }
                                }
                              }
                            }
                          }
                          frame True {
                            n342 = stacked-sequence {
                              tunnel: w466 -> [w475 w487 _]
                              frame #0 {
                                n343 = global read "Global.vi" "产品追溯码"() -> (w471:string)
                                "产品追溯码 2" <- w471
                                n344 = local read "productid"() -> (w470:string)
                                n345 = call "GetSQLstring.vi"("联机模式"=w475) -> ("错误输出"=w473:errorcluster, "连接字符串"=w474:string)  [unwired: 9 in]
                                n346 = Bundle("产品追溯码"=w471, "productid"=w470) -> (w469:cluster{"产品追溯码":string, "productid":string})  [unwired: 1 in]
                                n347 = call-poly <vilib>:"DB Tools Open Connection.vi"("error in (no error)"=w473, "connection information"=w474) -> ("error out"=w467:errorcluster, "connection reference"=w472:T9)  [unwired: 6 in]
                                n348 = Build Array(w469) -> (w468:cluster{"产品追溯码":string, "productid":string}[])
                                n349 = for {
                                tunnel: w472 -> [w481]
                                tunnel: w468 -> [w480] mode=indexing
                                shift-right: [w476] -> _
                                shift-left: w467 -> [w479]
                                n350 = call <vilib>:"DB Tools Insert Data.vi"("data"=w480, "error in (no error)"=w479, "columns"=string[] ["CODE_SENSOR", "PRODUCT_ID"], "table"="Code", "connection reference"=w481) -> ("error out"=w478:errorcluster)  [unwired: 5 in, 1 out]
                                n351 = case shown="无错误" w478 {
                                selector: w478 -> [w484 w486]
                                tunnel: [w484 w485] -> w477
                                frame No Error {
                                }
                                frame Error {
                                n352 = call <vilib>:"Clear Errors.vi"("error in (no error)"=w486) -> ("error out"=w485:errorcluster)  [unwired: 5 in, 1 out]
                                }
                                }
                                n353 = call <vilib>:"Simple Error Handler.vi"("error in (no error)"=w477) -> ("error out"=w476:errorcluster)  [unwired: 4 in, 4 out]
                                }
                              }
                              frame #1 {
                                n354 = global read "Global.vi" "产品追溯码"() -> (w488:string)
                                n355 = local read "productid"() -> (w496:string)
                                n356 = call "GetSQLstring.vi"("联机模式"=w487) -> ("错误输出"=w507:errorcluster, "连接字符串"=w508:string)  [unwired: 9 in]
                                n357 = Concatenate Strings("SELECT CODE_ID  FROM CODE  WHERE CODE_SENSOR ='" ("字符串"), w488, "'" ("字符串"), " AND PRODUCT_ID='" ("字符串"), w496, "'" ("字符串")) -> (w506:string)
                                n358 = call-poly <vilib>:"DB Tools Open Connection.vi"("error in (no error)"=w507, "connection information"=w508) -> ("error out"=w501:errorcluster, "connection reference"=w502:T9)  [unwired: 6 in]
                                n359 = call-poly <vilib>:"DB Tools Execute Query.vi"("error in (no error)"=w501, "SQL query"=w506, "connection reference"=w502) -> ("error out"=w504:errorcluster, "recordset reference"=w505:T10)  [unwired: 5 in]
                                n360 = call-poly <vilib>:"DB Tools Fetch Recordset Data.vi"("error in (no error)"=w504, "recordset reference"=w505) -> ("error out"=w500:errorcluster, "recordset data"=w503:variant[][])  [unwired: 3 in, 1 out]
                                n361 = Variant To Data(error in=w500, type=string[][] [], Variant=w503) -> (data=w499:string[][])  [unwired: 1 out]
                                n362 = Index Array(array=w499, index (row)=0 ("索引 (行)")) -> (element=w498:string[])  [unwired: 1 in]
                                n363 = Index Array(array=w498, index=0 ("索引 (行)")) -> (element=w497:string)
                                n364 = local write "codeid"(w497) -> ()
                              }
                              frame #2 {
                                n365 = global read "Global.vi" "上序状态颜色"() -> (w512:refnum<vi>)
                                n366 = local write "上序状态显示"("首序" ("上序状态显示")) -> ()
                                n367 = property class="Str"(reference=w512, "Value"="首序" ("上序状态显示")) -> (reference out=w510:refnum<vi>)  [unwired: 1 in, 1 out]
                                n368 = property on="上序状态" class="Bool (严格)"("Colors [4]"=cluster{u32, u32}[] [{6618880, 6618880}, {6618880, 6618880}, {6618880, 6618880}, {6618880, 6618880}]) -> ()  [unwired: 2 in, 2 out]
                                n369 = property class="Str"(reference=w510, "Text.BGColor"=u32 6618880) -> ()  [unwired: 1 in, 2 out]
                                n370 = call "设备状态.vi"("枚举"=enum16{"Read", "Write"}."Write", "Status_Write"=i16 2002) -> ()  [unwired: 9 in, 1 out]
                              }
                            }
                          }
                        }
                      }
                    }
                  }
                }
              }
            }
          }
          event "删除": Value Change {
            n371 = event-data() -> ("NewVal"=w517:bool)  [unwired: 1 in, 5 out]
            n372 = case shown="真" w517 {
              tunnel: w518 -> [_ w520]
              frame False {
              }
              frame True {
                n373 = Concatenate Strings("确认删除“", "请选择要删除的产品", "”吗？") -> (w522:string)
                n374 = Two Button Dialog(message=w522) -> (T button?=w521:bool)  [unwired: 2 in]
                n375 = case shown="真" w521 {
                  tunnel: w520 -> [_ w526]
                  tunnel: "请选择要删除的产品" -> [_ w525]
                  frame False {
                  }
                  frame True {
                    n376 = call <vilib>:"Open Config Data.vi"("configuration file path"=w526) -> ("error out"=w528:errorcluster, "refnum"=w531:T5)  [unwired: 8 in, 1 out]
                    n377 = call <vilib>:"Remove Section.vi"("section"=w525, "error in (no error)"=w528, "refnum"=w531) -> ("error out"=w530:errorcluster, "section exists?"=w527:bool, "refnum out"=w529:T5)  [unwired: 6 in]
                    n378 = case shown="假" w527 {
                      frame False {
                        n379 = One Button Dialog(message="删除失败！\n请确认产品存在！" ("消息")) -> ()  [unwired: 1 in, 1 out]
                      }
                      frame True {
                        n380 = One Button Dialog(message="删除成功！" ("消息")) -> ()  [unwired: 1 in, 1 out]
                      }
                    }
                    n381 = call <vilib>:"Close Config Data.vi"("error in (no error)"=w530, "refnum"=w529) -> ()  [unwired: 8 in, 2 out]
                  }
                }
              }
            }
          }
          event "确定": Value Change {
            n382 = event-data() -> ("NewVal"=w534:bool)  [unwired: 1 in, 5 out]
            n383 = case shown="真" w534 {
              frame False {
              }
              frame True {
                n384 = stacked-sequence {
                  seq-local: [w538 _ _ _ _ _ _ _] -> [_ _ _ _ _ _ _ _]
                  frame #0 {
                    n385 = global read "Global1.vi" "联机模式"() -> (w537:enum16{"单机", "追溯"})
                    n386 = case shown="\"追溯\"" w537 {
                      frame "单机", Default {
                      }
                      frame "追溯" {
                        n387 = local read "产品型号"() -> (w545:string)
                        n388 = call "Get_Device_ID.vi"() -> ("Device_ID"=→"deviceid":string)  [unwired: 10 in, 1 out]
                        n389 = call "GET_PRODUCT_ID.vi"("PRODFUCT_NAME"=w545) -> ("PRODUCT_ID"=w544:string)  [unwired: 10 in]
                        "productid" <- w544
                        n390 = call "查询前序设备.vi"("PRODUCT_ID"=w544) -> ("前序工位"=w543:string[])  [unwired: 10 in]
                        n391 = Index Array(array=w543, index=0 ("索引")) -> (element=→"Fdeviceid":string)
                      }
                    }
                    n392 = global read "Global.vi" "产品型号引用"() -> (w536:refnum<vi>)
                    n393 = local read "产品型号"() -> (w535:string)
                    "产品型号" <- w535
                    n394 = global write "Global1.vi" "产品型号"(w535) -> ()
                    n395 = property class="Str"(reference=w536, "Value"=w535) -> ()  [unwired: 1 in, 2 out]
                    n396 = String Subset(string=w535, offset (0)=u16 2 ("偏移量(0)"), length (rest)=u16 4 ("长度（剩余）")) -> (substring=w538:string)
                    n397 = Fract/Exp String To Number(string=w538) -> ()  [unwired: 3 in, 2 out]
                  }
                  frame #1 {
                    n398 = local read "用户名"() -> (w548:string)
                    n399 = global read "Global1.vi" "联机模式"() -> (w554:enum16{"单机", "追溯"})
                    n400 = call "GetSQLstring.vi"("联机模式"=w554) -> ("错误输出"=w556:errorcluster, "连接字符串"=w555:string)  [unwired: 9 in]
                    n401 = call-poly <vilib>:"DB Tools Open Connection.vi"("error in (no error)"=w556, "connection information"=w555) -> ("error out"=w562:errorcluster, "connection reference"=w561:T9)  [unwired: 6 in]
                    n402 = Concatenate Strings("SELECT USER_ID FROM [User]  WHERE USER_NAME ='", w548, "'" ("字符串")) -> (w557:string)
                    n403 = call-poly <vilib>:"DB Tools Execute Query.vi"("error in (no error)"=w562, "SQL query"=w557, "connection reference"=w561) -> ("error out"=w559:errorcluster, "recordset reference"=w558:T10)  [unwired: 5 in]
                    n404 = call-poly <vilib>:"DB Tools Fetch Recordset Data.vi"("error in (no error)"=w559, "recordset reference"=w558) -> ("error out"=w563:errorcluster, "recordset data"=w560:variant[][])  [unwired: 3 in, 1 out]
                    n405 = Variant To Data(error in=w563, type=string[][] [], Variant=w560) -> (data=w564:string[][])  [unwired: 1 out]
                    n406 = Index Array(array=w564, index (row)=0 ("索引 (行)")) -> (element=w565:string[])  [unwired: 1 in]
                    n407 = Index Array(array=w565, index=0 ("索引 (行)")) -> (element=→"USER_ID":string)
                  }
                  frame #2 {
                    n408 = local read "坐标轴参数"() -> (w579:string[][])
                    n409 = local read "结果判定参数"() -> (w574:string[][])
                    n410 = Index Array(array=w579, index (row) #1=0 ("索引 (行)"), index (row) #2=1 ("索引 (行)"), index (row) #3=2 ("索引 (行)"), index (row) #4=3 ("索引 (行)")) -> (element #1=w591:string[], element #2=w586:string[], element #3=w585:string[], element #4=w584:string[])  [unwired: 4 in]
                    n411 = Index Array(array=w591, index=1 ("索引")) -> (element=w583:string)
                    n412 = Index Array(array=w586, index=1 ("索引")) -> (element=w582:string)
                    n413 = Index Array(array=w585, index=1 ("索引")) -> (element=w581:string)
                    n414 = Index Array(array=w584, index=1 ("索引")) -> (element=w580:string)
                    n415 = for {
                      tunnel: w574 -> [w602] mode=indexing
                      tunnel: [w596] -> w571 mode=indexing
                      n416 = Index Array(array=w602) -> (element #1=w601:string, element #2=w600:string, element #3=w598:string)  [unwired: 3 in]
                      n417 = Fract/Exp String To Number(string=w600) -> (number=w599:dbl)  [unwired: 3 in, 1 out]
                      n418 = Fract/Exp String To Number(string=w598) -> (number=w597:dbl)  [unwired: 3 in, 1 out]
                      n419 = Bundle(w601, w599, w597) -> (w596:cluster{string, dbl, dbl})  [unwired: 1 in]
                    }
                    n420 = Fract/Exp String To Number(string=w583) -> (number=w578:dbl)  [unwired: 3 in, 1 out]
                    n421 = Fract/Exp String To Number(string=w582) -> (number=w577:dbl)  [unwired: 3 in, 1 out]
                    n422 = Fract/Exp String To Number(string=w581) -> (number=w576:dbl)  [unwired: 3 in, 1 out]
                    n423 = Fract/Exp String To Number(string=w580) -> (number=w575:dbl)  [unwired: 3 in, 1 out]
                    n424 = property on="力位移曲线 3" class="XYGraph (严格)"("XScale.Minimum"=w578) -> ()  [unwired: 2 in, 2 out]
                    n425 = property on="力位移曲线 3" class="XYGraph (严格)"("XScale.Maximum"=w577) -> ()  [unwired: 2 in, 2 out]
                    n426 = property on="力位移曲线 3" class="XYGraph (严格)"("YScale.Minimum"=w576) -> ()  [unwired: 2 in, 2 out]
                    n427 = property on="力位移曲线 3" class="XYGraph (严格)"("YScale.Maximum"=w575) -> ()  [unwired: 2 in, 2 out]
                    n428 = Index Array(array=w571, index #3=3 ("索引")) -> (element #1=w569:cluster{string, dbl, dbl}, element #2=w568:cluster{string, dbl, dbl}, element #3=w567:cluster{string, dbl, dbl})  [unwired: 2 in]
                    n429 = Array To Cluster(array=w571) -> (cluster=w572:T11)
                    n430 = Build Array(w569, w568, w567) -> (w566:cluster{string, dbl, dbl}[])
                    n431 = Array To Cluster(array=w566) -> (cluster=w573:T12)
                    n432 = global write "Global.vi" "复检判定参数"(w572) -> ()
                    n433 = global write "Global.vi" "最大值判定参数"(w573) -> ()
                  }
                  frame #3 {
                    n434 = local read "判定框参数"() -> (w612:string[][])
                    n435 = Index Array(array=w612, index (row) #1=0 ("索引 (行)"), index (row) #2=0 ("索引 (行)"), index (row) #3=1 ("索引 (行)"), index (row) #4=1 ("索引 (行)")) -> (element #1=w620:string[], element #2=w615:string[], element #3=w614:string[], element #4=w613:string[])  [unwired: 4 in]
                    n436 = Index Array(array=w620, index=1 ("索引")) -> (element=w607:string)
                    n437 = Index Array(array=w615, index=2 ("索引")) -> (element=w606:string)
                    n438 = Index Array(array=w614, index=1 ("索引")) -> (element=w605:string)
                    n439 = Index Array(array=w613, index=2 ("索引")) -> (element=w604:string)
                    n440 = local read "力位移曲线 3"() -> (w625:cluster{dbl[], dbl[]}[])
                    n441 = Fract/Exp String To Number(string=w607) -> (number=w611:dbl)  [unwired: 3 in, 1 out]
                    n442 = Fract/Exp String To Number(string=w606) -> (number=w610:dbl)  [unwired: 3 in, 1 out]
                    n443 = Fract/Exp String To Number(string=w605) -> (number=w608:dbl)  [unwired: 3 in, 1 out]
                    n444 = Fract/Exp String To Number(string=w604) -> (number=w609:dbl)  [unwired: 3 in, 1 out]
                    n445 = for {
                      tunnel: [w632] -> w603 mode=indexing
                      tunnel: w625 -> [w631] mode=indexing
                      tunnel: w611 -> [w629]
                      tunnel: w610 -> [w628]
                      tunnel: w609 -> [w627]
                      tunnel: w608 -> [w626]
                      i -> [w630]
                      n446 = case shown="0" w630 {
                        tunnel: [w633 w638] -> w632
                        tunnel: w631 -> [w633 _]
                        tunnel: w629 -> [_ w637]
                        tunnel: w628 -> [_ w636]
                        tunnel: w627 -> [_ w635]
                        tunnel: w626 -> [_ w634]
                        frame Default {
                        }
                        frame 0 {
                          n447 = Build Array(w637, w637, w636, w636, w637) -> (w639:dbl[])
                          n448 = Build Array(w634, w635, w635, w634, w634) -> (w640:dbl[])
                          n449 = Bundle(w639, w640) -> (w638:cluster{dbl[], dbl[]})  [unwired: 1 in]
                        }
                      }
                    }
                    n450 = local write "力位移曲线 3"(w603) -> ()
                  }
                  frame #4 {
                    n451 = local read "判定框参数"() -> (w641:string[][])
                    n452 = Index Array(array=w641, index (row) #1=2 ("索引 (行)"), index (row) #2=2 ("索引 (行)"), index (row) #3=3 ("索引 (行)"), index (row) #4=3 ("索引 (行)")) -> (element #1=w659:string[], element #2=w654:string[], element #3=w653:string[], element #4=w652:string[])  [unwired: 4 in]
                    n453 = Index Array(array=w659, index=1 ("索引")) -> (element=w647:string)
                    n454 = Index Array(array=w654, index=2 ("索引")) -> (element=w646:string)
                    n455 = Index Array(array=w653, index=1 ("索引")) -> (element=w645:string)
                    n456 = Index Array(array=w652, index=2 ("索引")) -> (element=w644:string)
                    n457 = local read "力位移曲线 3"() -> (w642:cluster{dbl[], dbl[]}[])
                    n458 = Fract/Exp String To Number(string=w647) -> (number=w651:dbl)  [unwired: 3 in, 1 out]
                    n459 = Fract/Exp String To Number(string=w646) -> (number=w650:dbl)  [unwired: 3 in, 1 out]
                    n460 = Fract/Exp String To Number(string=w645) -> (number=w648:dbl)  [unwired: 3 in, 1 out]
                    n461 = Fract/Exp String To Number(string=w644) -> (number=w649:dbl)  [unwired: 3 in, 1 out]
                    n462 = for {
                      tunnel: [w670] -> w643 mode=indexing
                      tunnel: w642 -> [w669] mode=indexing
                      tunnel: w651 -> [w667]
                      tunnel: w650 -> [w666]
                      tunnel: w649 -> [w665]
                      tunnel: w648 -> [w664]
                      i -> [w668]
                      n463 = case shown="1" w668 {
                        tunnel: [w671 w676] -> w670
                        tunnel: w669 -> [w671 _]
                        tunnel: w667 -> [_ w675]
                        tunnel: w666 -> [_ w674]
                        tunnel: w665 -> [_ w673]
                        tunnel: w664 -> [_ w672]
                        frame Default {
                        }
                        frame 1 {
                          n464 = Build Array(w675, w675, w674, w674, w675) -> (w677:dbl[])
                          n465 = Build Array(w672, w673, w673, w672, w672) -> (w678:dbl[])
                          n466 = Bundle(w677, w678) -> (w676:cluster{dbl[], dbl[]})  [unwired: 1 in]
                        }
                      }
                    }
                    n467 = local write "力位移曲线 3"(w643) -> ()
                  }
                  frame #5 {
                    n468 = local read "结果判定参数"() -> (w692:string[][])
                    n469 = Index Array(array=w692, index (row) #1=0 ("索引 (行)"), index (row) #2=0 ("索引 (行)"), index (row) #3=1 ("索引 (行)"), index (row) #4=1 ("索引 (行)")) -> (element #1=w700:string[], element #2=w699:string[], element #3=w698:string[], element #4=w697:string[])  [unwired: 4 in]
                    n470 = Index Array(array=w700, index=1 ("索引")) -> (element=w696:string)
                    n471 = Index Array(array=w699, index=2 ("索引")) -> (element=w695:string)
                    n472 = Index Array(array=w698, index=1 ("索引")) -> (element=w694:string)
                    n473 = Index Array(array=w697, index=2 ("索引")) -> (element=w693:string)
                    n474 = Fract/Exp String To Number(string=w696) -> (number=→"最大值上限":dbl)  [unwired: 3 in, 1 out]
                    n475 = Fract/Exp String To Number(string=w695) -> (number=→"最大值下限":dbl)  [unwired: 3 in, 1 out]
                    n476 = Fract/Exp String To Number(string=w694) -> (number=→"最小值上限":dbl)  [unwired: 3 in, 1 out]
                    n477 = Fract/Exp String To Number(string=w693) -> (number=→"最小值下限":dbl)  [unwired: 3 in, 1 out]
                    n478 = property on="选项卡控件 2" class="TabCtl (严格)"("Value"=enum32{"滑移力曲线", "参数查看"}."滑移力曲线" ("选项卡控件 2")) -> ()  [unwired: 2 in, 2 out]
                  }
                  frame #6 {
                    n479 = local read "产品型号"() -> (w701:string)
                    n480 = case shown="\"R128\", 默认" w701 {
                      frame "R092B" {
                        w702 = FALSE
                        n481 = property on="最小值下限" class="DigNum (严格)"("Visible"=w702) -> ()  [unwired: 2 in, 2 out]
                        n482 = property on="最小值上限" class="DigNum (严格)"("Visible"=w702) -> ()  [unwired: 2 in, 2 out]
                        n483 = property on="压位移内最小压力(N)" class="DigNum (严格)"("Visible"=w702) -> ()  [unwired: 2 in, 2 out]
                        n484 = property on="拉位移内最小压力(N)" class="DigNum (严格)"("Visible"=w702) -> ()  [unwired: 2 in, 2 out]
                      }
                      frame "R567X" {
                        w703 = FALSE
                        n485 = property on="最小值下限" class="DigNum (严格)"("Visible"=w703) -> ()  [unwired: 2 in, 2 out]
                        n486 = property on="最小值上限" class="DigNum (严格)"("Visible"=w703) -> ()  [unwired: 2 in, 2 out]
                        n487 = property on="压位移内最小压力(N)" class="DigNum (严格)"("Visible"=w703) -> ()  [unwired: 2 in, 2 out]
                        n488 = property on="拉位移内最小压力(N)" class="DigNum (严格)"("Visible"=w703) -> ()  [unwired: 2 in, 2 out]
                      }
                      frame "R563X" {
                        w704 = FALSE
                        n489 = property on="最小值下限" class="DigNum (严格)"("Visible"=w704) -> ()  [unwired: 2 in, 2 out]
                        n490 = property on="最小值上限" class="DigNum (严格)"("Visible"=w704) -> ()  [unwired: 2 in, 2 out]
                        n491 = property on="压位移内最小压力(N)" class="DigNum (严格)"("Visible"=w704) -> ()  [unwired: 2 in, 2 out]
                        n492 = property on="拉位移内最小压力(N)" class="DigNum (严格)"("Visible"=w704) -> ()  [unwired: 2 in, 2 out]
                      }
                      frame "R128", Default {
                        w705 = FALSE
                        n493 = property on="最小值下限" class="DigNum (严格)"("Visible"=w705) -> ()  [unwired: 2 in, 2 out]
                        n494 = property on="最小值上限" class="DigNum (严格)"("Visible"=w705) -> ()  [unwired: 2 in, 2 out]
                        n495 = property on="压位移内最小压力(N)" class="DigNum (严格)"("Visible"=w705) -> ()  [unwired: 2 in, 2 out]
                        n496 = property on="拉位移内最小压力(N)" class="DigNum (严格)"("Visible"=w705) -> ()  [unwired: 2 in, 2 out]
                      }
                    }
                  }
                  frame #7 {
                    w706 = "参数装载成功！" ("消息")
                    n497 = call "浮动通知.vi"("通知内容"=w706) -> ()  [unwired: 11 in]
                    n498 = One Button Dialog(message=w706) -> ()  [unwired: 1 in, 1 out]
                  }
                }
              }
            }
          }
          event "添加": Value Change {
            n499 = event-data() -> ("NewVal"=w709:bool)  [unwired: 1 in, 5 out]
            n500 = local read "请输入添加的产品名称"() -> (w710:string)
            n501 = call <vilib>:"Trim Whitespace.vi"("string"=w710) -> ("trimmed string"=w711:string)  [unwired: 1 in]
            n502 = White Space?(1:w711) -> (0:w712:bool)
            n503 = case shown="假" w712 {
              tunnel: w707 -> [w715 _]
              tunnel: w709 -> [w714 _]
              tunnel: w708 -> [w713 _]
              frame False {
                n504 = case shown="真" w714 {
                  tunnel: w715 -> [_ w717]
                  tunnel: w713 -> [_ w716]
                  frame False {
                  }
                  frame True {
                    n505 = for {
                      tunnel: w717 -> [w720] mode=indexing
                      tunnel: w716 -> [w719]
                      n506 = call "Read_Write ParaINI File.vi"("Mode"=enum16{"Read", "Write"}."Write", "Section"="请输入添加的产品名称", "Filepath"=w719, "Ctl Refnum"=w720) -> ()  [unwired: 7 in, 1 out]
                    }
                  }
                }
              }
              frame True {
                w722 = 64 items=["None"=0, "Hand, Error, Stop"=16, "Question"=32, "Exclamation, Warning"=48, "Asterisk, Information"=64] ("icon")
                w723 = 0 items=["OK", "OKCancel", "AbortRetryIgnore", "YesNoCancel", "YesNo", "RetryCancel"] ("buttons")
                n507 = call "信息框（标题、文本、图标）.vi"("icon"=w722, "buttons"=w723, "caption"="添加失败", "text"="请输入产品名称!") -> ()  [unwired: 6 in, 2 out]
              }
            }
          }
          event "产品型号": Value Change {
            n508 = event-data() -> ()  [unwired: 1 in, 6 out]
            n509 = stacked-sequence {
              tunnel: w726 -> [_ w729]
              tunnel: w727 -> [_ w728]
              frame #0 {
              }
              frame #1 {
                n510 = for {
                  tunnel: w729 -> [w732] mode=indexing
                  tunnel: w728 -> [w731]
                  n511 = local read "产品型号"() -> (w730:string)
                  n512 = call "Read_Write ParaINI File.vi"("Mode"=enum16{"Read", "Write"}."Read", "Section"=w730, "Filepath"=w731, "Ctl Refnum"=w732) -> ()  [unwired: 7 in, 1 out]
                }
              }
            }
          }
          event "退出": Value Change {
            n513 = event-data() -> ()  [unwired: 1 in, 6 out]
            n514 = control-ref of="本VI"() -> (w736:refnum<vi>)
            n515 = invoke class="VI" method="FP.Close"(reference=w736) -> (reference out=w734:refnum<vi>, error out=w735:errorcluster)  [unwired: 2 in, 1 out]
            n516 = Close Reference(reference=w734, error in (no error)=w735) -> ()  [unwired: 1 out]
          }
          event "更新": Value Change {
            n517 = event-data() -> ("NewVal"=w739:bool)  [unwired: 1 in, 5 out]
            n518 = case shown="真" w739 {
              tunnel: w738 -> [_ w742]
              tunnel: w737 -> [_ w741]
              frame False {
              }
              frame True {
                n519 = for {
                  tunnel: w742 -> [w747]
                  tunnel: w741 -> [w746] mode=indexing
                  tunnel: [w745] -> w740
                  n520 = local read "产品型号"() -> (w749:string)
                  n521 = call "Read_Write ParaINI File.vi"("Mode"=enum16{"Read", "Write"}."Write", "Section"=w749, "Filepath"=w747, "Ctl Refnum"=w746) -> ("error out"=w745:errorcluster)  [unwired: 7 in]
                }
                n522 = case shown="无错误" w740 {
                  frame No Error {
                    n523 = call "浮动通知.vi"("通知内容"="更新成功！") -> ()  [unwired: 11 in]
                  }
                  frame Error {
                    n524 = call "浮动通知.vi"("通知内容"="更新失败！") -> ()  [unwired: 11 in]
                  }
                }
              }
            }
          }
          event "请输入添加的产品名称": Value Change {
            n525 = event-data() -> ("NewVal"=w750:string)  [unwired: 1 in, 5 out]
            n526 = control-ref of="产品型号"() -> (w751:refnum<vi>)
            n527 = property on="属性节点" class="CmbBox"(reference=w751) -> ("Strings[]"=w752:string[])  [unwired: 1 in, 2 out]
            n528 = for {
              tunnel: w750 -> [w753]
              tunnel: w752 -> [w754] mode=indexing
              n529 = Equal?(x=w753, y=w754) -> (x = y?=w755:bool)
              n530 = case shown="真" w755 {
                tunnel: w753 -> [_ w756]
                frame False {
                }
                frame True {
                  n531 = stacked-sequence {
                    tunnel: w756 -> [w762 _]
                    frame #0 {
                      w757 = 64 items=["None"=0, "Hand, Error, Stop"=16, "Question"=32, "Exclamation, Warning"=48, "Asterisk, Information"=64] ("icon")
                      w758 = 0 items=["OK", "OKCancel", "AbortRetryIgnore", "YesNoCancel", "YesNo", "RetryCancel"] ("buttons")
                      n532 = Concatenate Strings("已经存在产品”" ("text"), w762, "“\n请勿重复添加！" ("字符串")) -> (w760:string)
                      n533 = call "信息框（标题、文本、图标）.vi"("icon"=w757, "buttons"=w758, "caption"="产品重复", "text"=w760) -> ()  [unwired: 6 in, 2 out]
                    }
                    frame #1 {
                      n534 = local write "请输入添加的产品名称"("" ("请输入添加的产品名称")) -> ()
                    }
                  }
                }
              }
            }
          }
          event Panel Close? {
            n535 = event-data() -> ()  [unwired: 1 in, 4 out]
            n536 = control-ref of="本VI"() -> (w769:refnum<vi>)
            n537 = invoke class="VI" method="Abort VI"(reference=w769) -> (reference out=w766:refnum<vi>, error out=w765:errorcluster)  [unwired: 2 in, 1 out]
            n538 = invoke class="VI" method="FP.Close"(reference=w766, error in=w765) -> (reference out=w767:refnum<vi>, error out=w768:errorcluster)  [unwired: 1 in, 1 out]
            n539 = Close Reference(reference=w767, error in (no error)=w768) -> ()  [unwired: 1 out]
            n540 = global write "Global.vi" "程序关闭"(TRUE ("程序关闭")) -> ()
            n541 = event-data("Discard?"=TRUE ("放弃？")) -> ()  [unwired: 1 in, 1 out]
          }
          event "进入用户管理": Value Change {
            n542 = event-data() -> ()  [unwired: 1 in, 6 out]
            n543 = vi-ref "User_manager.vi"() -> (w773:refnum<vi>)
            n544 = call "CallVI.vi"("VI引用"=w773, "状态"=T1."Maximized") -> ()  [unwired: 12 in, 2 out]
          }
          event "设备故障": Value Change {
            n545 = event-data() -> ()  [unwired: 1 in, 6 out]
            n546 = call "状态改变.vi"("设备状态"=enum16{"设备离线", "设备正常", "设备缺料", "设备故障", "质量报警"}."设备故障") -> ()  [unwired: 11 in]
          }
          event "设备缺料": Value Change {
            n547 = event-data() -> ()  [unwired: 1 in, 6 out]
            n548 = call "状态改变.vi"("设备状态"=enum16{"设备离线", "设备正常", "设备缺料", "设备故障", "质量报警"}."设备缺料") -> ()  [unwired: 11 in]
          }
          event "质量报警": Value Change {
            n549 = event-data() -> ()  [unwired: 1 in, 6 out]
            n550 = call "状态改变.vi"("设备状态"=enum16{"设备离线", "设备正常", "设备缺料", "设备故障", "质量报警"}."质量报警") -> ()  [unwired: 11 in]
          }
        }
        n551 = global read "Global.vi" "程序关闭"() -> (w118:bool)
      }
    }
  }
